vi "Handle Error.vi"(8 "error in (no error)":errorcluster, 11 "Server in":refnum<class "Server.lvclass">) -> (0 "error out":errorcluster, 2 "stop actor?":bool=TRUE, 3 "Server out":refnum<class "Server.lvclass">)   [LabVIEW 2021, in "Server.lvlib" / "Server.lvclass"]
doc: "(<B>Filename</B>: Actor Framework.lvlib:Actor.lvclass:Handle Error.vi)\n\nDefines how the actor handles an error that occurred while processing a message. By default, this method does nothing except stop the actor."
uses:
  Server.lvclass
  <vilib>/ActorFramework/Actor/Actor.lvclass
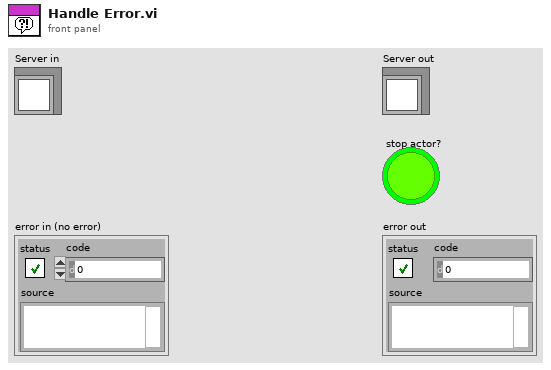
[diagram p1: front panel]
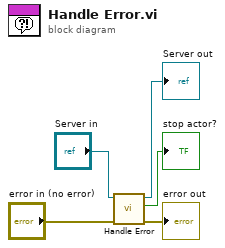
[diagram p0: block diagram]
diagram:
  n1 = call-parent "Handle Error.vi"("error in (no error)"="error in (no error)", "Actor in"="Server in") -> ("error out"=→"error out":errorcluster, "stop actor?"=→"stop actor?":bool, "Actor out"=→"Server out":refnum<class "Server.lvclass">)  [unwired: 7 in]
